vi "Execute.vi"(8 "error in (no error)":errorcluster, 9 "System in":refnum<class "System.lvclass">, 10 "Command in":refnum<class "Command.lvclass">, 11 "DMD-DFD-Driving-State in":refnum<class "DMD-DFD-Driving-State.lvclass">) -> (0 "error out":errorcluster, 2 "Next State":refnum<class "State.lvclass">, 3 "DMD-DFD-Driving-State out":refnum<class "DMD-DFD-Driving-State.lvclass">)   [LabVIEW 2013, in "DMD-DFD-Driving-State.lvclass"]
uses:
  DMD-DFD-Driving-State.lvclass
  Commands/Command/Command.lvclass
  Systems/System/System.lvclass
  State/State.lvclass
  Systems/DriveMotors/DriveMotors.lvclass
  Commands/DM-DriveForwardDistance/DM-DriveForwardDistance.lvclass
  DM-DFD-StopAtDistance-State/DM-DFD-StopAtDistance-State.lvclass
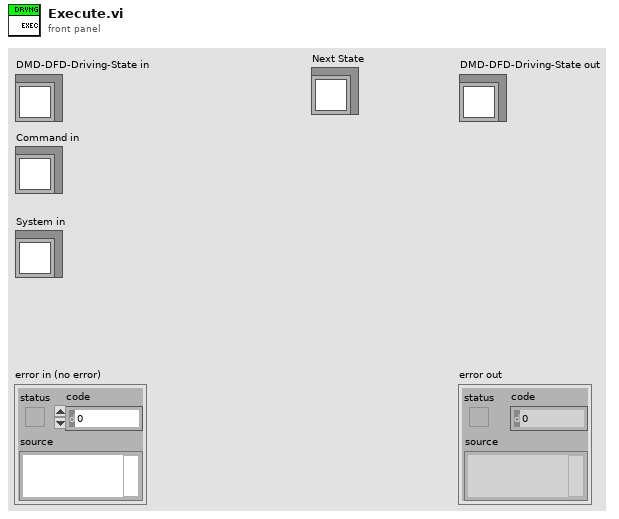
[diagram p1: front panel]
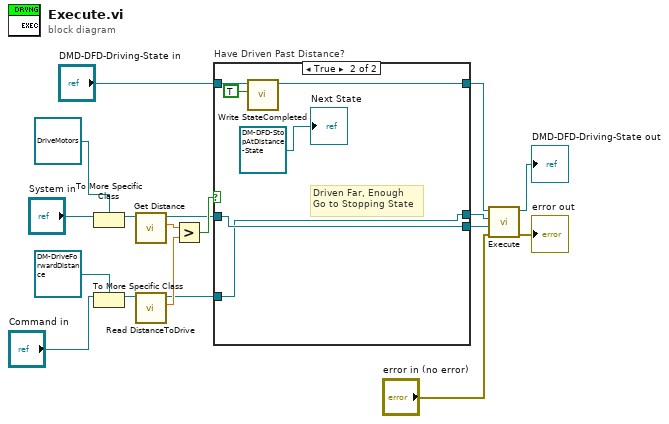
[diagram p0: block diagram]
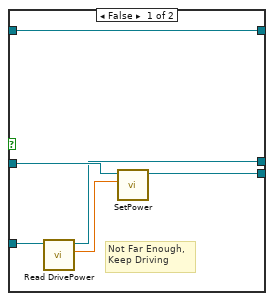
[diagram p2: hidden frame]
diagram:
  n1 = To More Specific Class(target class=refnum<class "DriveMotors.lvclass"> refnum ("DriveMotors.lvclass"), reference="System in") -> (specific class reference=w10:refnum<class "DriveMotors.lvclass">)  [unwired: 1 in, 1 out]
  n2 = To More Specific Class(target class=refnum<class "DM-DriveForwardDistance.lvclass"> refnum ("DM-DriveForwardDistance.lvclass"), reference="Command in") -> (specific class reference=w11:refnum<class "DM-DriveForwardDistance.lvclass">)  [unwired: 1 in, 1 out]
  n3 = call-dynamic "Get Distance.vi"("DriveMotors in"=w10) -> ("Distance"=w9:dbl, "DriveMotors out"=w6:refnum<class "DriveMotors.lvclass">)  [unwired: 8 in, 1 out]
  n4 = call-dynamic "Read DistanceToDrive.vi"("DM-DriveForwardDistance in"=w11) -> ("DistanceToDrive"=w8:dbl, "DM-DriveForwardDistance out"=w4:refnum<class "DM-DriveForwardDistance.lvclass">)  [unwired: 8 in, 1 out]
  n5 = Greater?(x=w9, y=w8) -> (0:w7:bool)
  n6 = case "Have Driven Past Distance?" shown="True" w7 {
    tunnel: w6 -> [w24 w29]
    tunnel: [w23 w29] -> w5
    tunnel: w4 -> [w22 w28]
    tunnel: [w20 w28] -> w3
    tunnel: "DMD-DFD-Driving-State in" -> [w19 w27]
    tunnel: [w19 w26] -> w1
    frame False {
      # "Not Far Enough,\nKeep Driving"
      # "Not Far Enough, Keep Going"
      n7 = call-dynamic "Read DrivePower.vi"("DM-DriveForwardDistance in"=w22) -> ("DrivePower"=w21:dbl, "DM-DriveForwardDistance out"=w20:refnum<class "DM-DriveForwardDistance.lvclass">)  [unwired: 8 in, 1 out]
      n8 = call-dynamic "SetPower.vi"("MotorPower"=w21, "DriveMotors in"=w24) -> ("DriveMotors out"=w23:refnum<class "DriveMotors.lvclass">)  [unwired: 8 in, 1 out]
    }
    frame True {
      # "Driven Far, Enough\nGo to Stopping State"
      # "Yes, So go to Stop At Distance"
      n9 = call-dynamic "Write StateCompleted.vi"("StateCompleted"=TRUE, "State in"=w27) -> ("State out"=w26:refnum<class "DMD-DFD-Driving-State.lvclass">)  [unwired: 8 in, 1 out]
      "Next State" <- refnum<class "DM-DFD-StopAtDistance-State.lvclass"> refnum ("DM-DFD-StopAtDistance-State.lvclass")
    }
  }
  n10 = call-parent "Execute.vi"("error in (no error)"="error in (no error)", "System in"=w5, "Command in"=w3, "State in"=w1) -> ("error out"=→"error out":errorcluster, "State out"=→"DMD-DFD-Driving-State out":refnum<class "DMD-DFD-Driving-State.lvclass">)  [unwired: 5 in, 1 out]
